vi "HandShaking.vi"(6 "Elapsed Time":u32, 8 "error in (no error)":errorcluster, 10 "Event Sources":T1, 11 "TestExec in":refnum<class "TestExec.lvclass">) -> (0 "error out":errorcluster, 3 "TestExec out":refnum<class "TestExec.lvclass">)   [LabVIEW 2021, in "OPC UA.lvlib" / "TestExec.lvclass"]
uses:
  TestExec.lvclass
  TestExec.lvclass/TestExec.ctl
  a96ab253-98d7-4f61-9cc2-4ba11fd792e5.vi
  <vilib>/addons/TestStand/_TSUtility.llb/TestStand - Get Property Value (Boolean).vi
  <vilib>/addons/TestStand/_TSUtility.llb/TestStand - Get Property Value (Number {Signed 32-bit Integer}).vi
  <vilib>/addons/TestStand/_TSUtility.llb/TestStand - Set Property Value (Boolean).vi
  OPC UA/OPC UA.lvclass
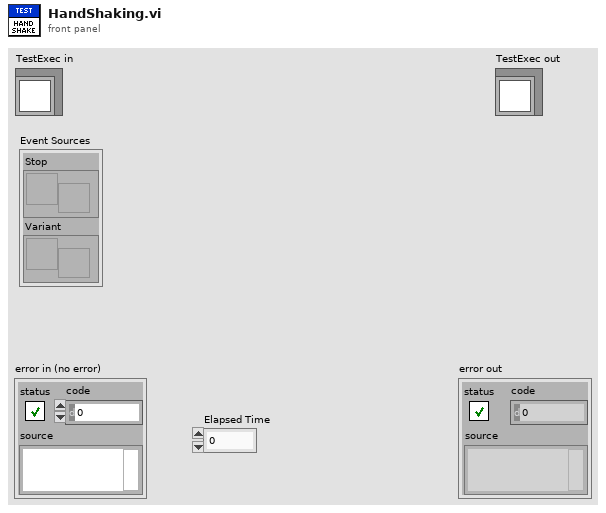
[diagram p1: front panel]
types:
  T1 = cluster{"Stop":refnum<user-event>, "Variant":refnum<user-event>}
  T2 = typedef "TestExec.lvclass/Rx TestExec.ctl" = cluster{"Cylinder_1":bool, "Cylinder_2":bool, "Cylinder_3":bool, "Cylinder_4":bool, "Cylinder_5":bool, "StepEcho":u32, "Reset":bool, "Stop":bool, "FaultCode":u32}
  T3 = typedef "OPC UA.lvlib/TestExec.lvclass/Tx TestExec.ctl" = cluster{"HighVoltage":bool, "TestRunning":bool, "StepNo":u32, "Fault":bool, "Heartbeat":bool}
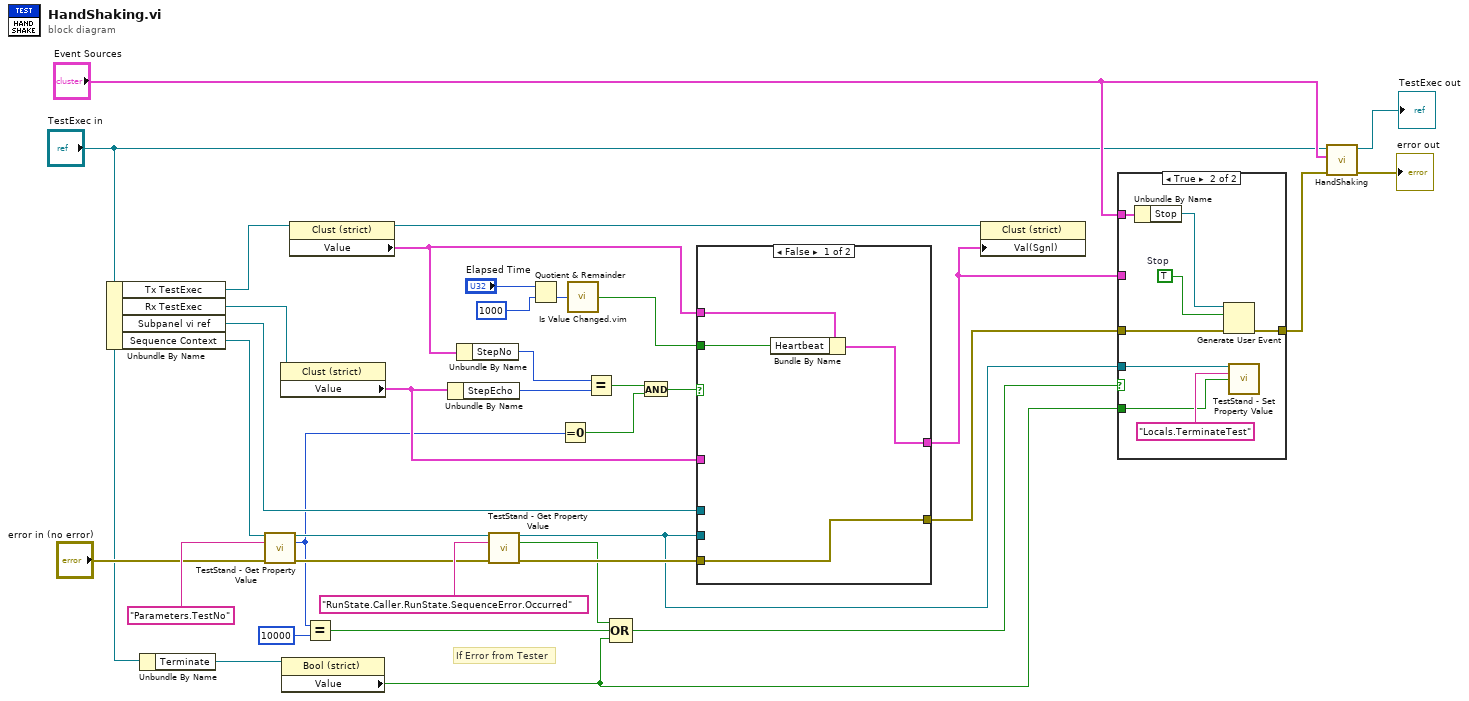
[diagram p0: block diagram]
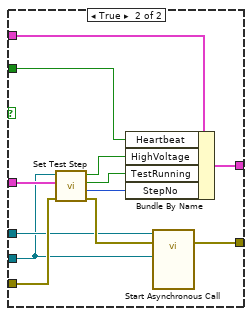
[diagram p2: hidden frame]
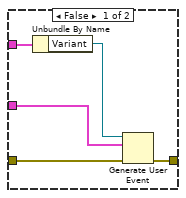
[diagram p3: hidden frame]
diagram:
  # "If Error from Tester"
  n1 = Unbundle By Name("TestExec in") -> ("Tx TestExec"=w34:refnum<vi>, "Rx TestExec"=w36:refnum<vi>, "Subpanel vi ref"=w29:refnum<vi>, "Sequence Context"=w20:refnum<k7>)
  n2 = Unbundle By Name("TestExec in") -> ("Terminate"=w11:refnum<vi>)
  n3 = call-poly <vilib>:"TestStand - Get Property Value.vi"("Sequence Context In"=w20, "Lookup String"="Parameters.TestNo" ("Test Number"), "error in (no error)"="error in (no error)") -> ("Sequence Context Out"=w19:refnum<k7>, "Value"=w6:i32, "error out"=w18:errorcluster)  [unwired: 10 in]
  n4 = property on="Property Node" class="Clust (strict)"(reference=w36) -> ("Value"=w28:T2)  [unwired: 1 in, 2 out]
  n5 = property on="Property Node" class="Bool (strict)"(reference=w11) -> ("Value"=w10:bool)  [unwired: 1 in, 2 out]
  n6 = property on="Property Node" class="Clust (strict)"(reference=w34) -> (reference out=w2:refnum<vi>, "Value"=w9:T3)  [unwired: 1 in, 1 out]
  n7 = Equal?(x=w6, y=10000 ("x")) -> (x = y?=w4:bool)
  n8 = Unbundle By Name(w28) -> ("StepEcho"=w32:u32)
  n9 = Unbundle By Name(w9) -> ("StepNo"=w33:u32)
  n10 = call-poly <vilib>:"TestStand - Get Property Value.vi"("Sequence Context In"=w19, "Lookup String"="RunState.Caller.RunState.SequenceError.Occurred", "error in (no error)"=w18) -> ("Sequence Context Out"=w12:refnum<k7>, "Value"=w5:bool, "error out"=w31:errorcluster)  [unwired: 10 in]
  n11 = Quotient & Remainder(x="Elapsed Time", y=u32 1000) -> (floor(x/y)=w24:u32)  [unwired: 1 out]
  n12 = Equal To 0?(x=w6) -> (x = 0?=w14:bool)
  n13 = call "Is Value Changed.vim"("value"=w24) -> ("changed or first call?"=w3:bool)
  n14 = Equal?(x=w33, y=w32) -> (x = y?=w16:bool)
  n15 = Compound Arithmetic op=OR(w5, w4, w10) -> (w8:bool)
  n16 = And(x=w16, y=w14) -> (x .and. y?=w15:bool)
  n17 = case shown="False" w15 {
    tunnel: w28 -> [_ w53]
    tunnel: w31 -> [w41 w52]
    tunnel: [w41 w46] -> w27
    tunnel: w9 -> [w40 w47]
    tunnel: w12 -> [_ w44]
    tunnel: w29 -> [_ w45]
    tunnel: w3 -> [w39 w43]
    tunnel: [w38 w42] -> w1
    frame False {
      n18 = Bundle By Name(cluster=w40, "Heartbeat"=w39) -> (w38:T3)
    }
    frame True {
      n19 = call "Set Test Step .vi"("error in (no error)"=w52, "Rx Tester"=w53, "Sequence Context In"=w44) -> ("error out"=w48:errorcluster, "Next Step"=w49:i32, "Test Running"=w50:bool, "HV"=w51:bool)  [unwired: 5 in]
      n20 = Bundle By Name(cluster=w47, "Heartbeat"=w43, "HighVoltage"=w51, "TestRunning"=w50, "StepNo"=w49) -> (w42:T3)
      n21 = call-by-ref "Start Asynchronous Call"(reference=w45, error in=w48, "Sequence Context"=w44) -> (error out=w46:errorcluster)  [unwired: 10 in, 2 out]
    }
  }
  n22 = property on="Property Node" class="Clust (strict)"(reference=w2, "Val(Sgnl)"=w1) -> ()  [unwired: 1 in, 2 out]
  n23 = case shown="True" w8 {
    tunnel: w1 -> [w58 _]
    tunnel: "Event Sources" -> [w57 w66]
    tunnel: w27 -> [w55 w63]
    tunnel: [w54 w62] -> w26
    tunnel: w12 -> [_ w61]
    tunnel: w10 -> [_ w59]
    frame False {
      n24 = Unbundle By Name(w57) -> ("Variant"=w56:refnum<user-event>)
      n25 = Generate User Event(user event=w56, event data cluster=w58, error in=w55) -> (error out=w54:errorcluster)  [unwired: 1 in, 1 out]
    }
    frame True {
      w64 = TRUE  # Stop
      n26 = Unbundle By Name(w66) -> ("Stop"=w65:refnum<user-event>)
      n27 = Generate User Event(user event=w65, event data cluster=w64, error in=w63) -> (error out=w62:errorcluster)  [unwired: 1 in, 1 out]
      n28 = call-poly <vilib>:"TestStand - Set Property Value.vi"("Sequence Context In"=w61, "Lookup String"="Locals.TerminateTest", "New Value"=w59) -> ()  [unwired: 11 in, 2 out]
    }
  }
  n29 = call-parent "HandShaking.vi"("error in (no error)"=w26, "Event Sources"="Event Sources", "OPC UA in"="TestExec in") -> ("error out"=→"error out":errorcluster, "OPC UA out"=→"TestExec out":refnum<class "TestExec.lvclass">)  [unwired: 7 in]
